vi "Accurate Measure_BU2.vi"(0 "DMM ref in":refnum<visa-resource-name>, 1 "channel_count":i32=11, 2 "P_current_count":i32, 3 "N_current_count":i32, 5 "DMM error in":errorcluster, 7 "Enable DMM-\nRelay":bool=TRUE, 9 "ESP32 ref in":refnum<visa-resource-name>, 11 "ESP32 error in":errorcluster, 12 "current_mode":u8[](array[numeric])=[0, 0, 0, 0, 0, 0, 0, 0, 0, 0, 0]) -> (4 "DMM ref out":refnum<visa-resource-name>, 6 "DMM error out":errorcluster, 8 "Accurate Data":dbl[](array[numeric]), 10 "ESP32 ref out":refnum<visa-resource-name>, 13 "time_out_count":i32, 14 "Standard Deviation of Data":dbl[](array[numeric]), 15 "ESP32 error out":errorcluster)   [LabVIEW 2023]
uses:
  <instrlib>/Agilent 3446X Series/Agilent 3446X Series.lvlib
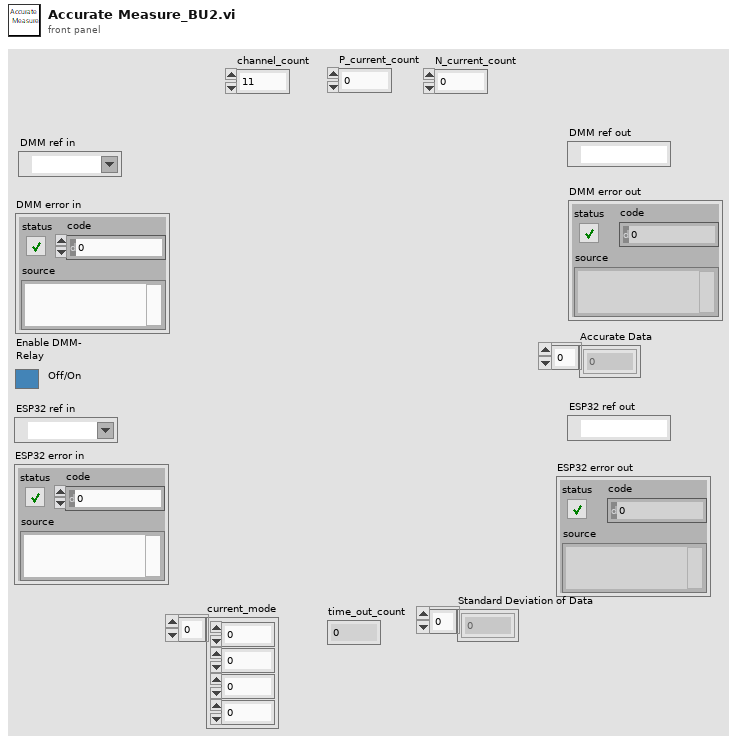
[diagram p1: front panel]
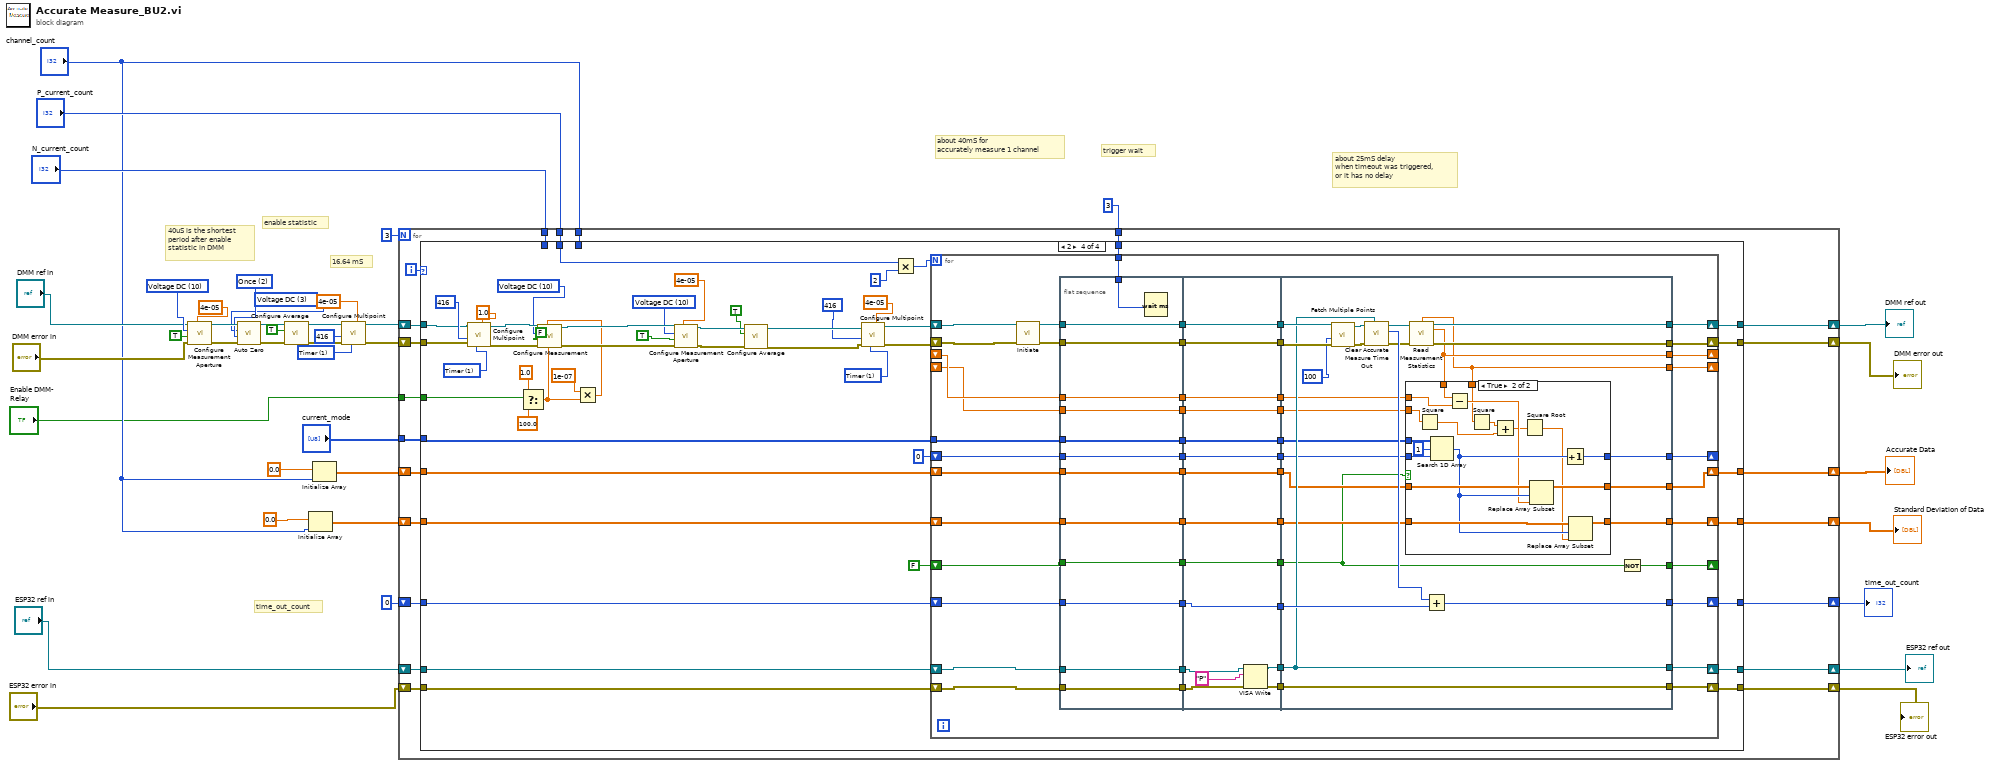
[diagram p0: block diagram]
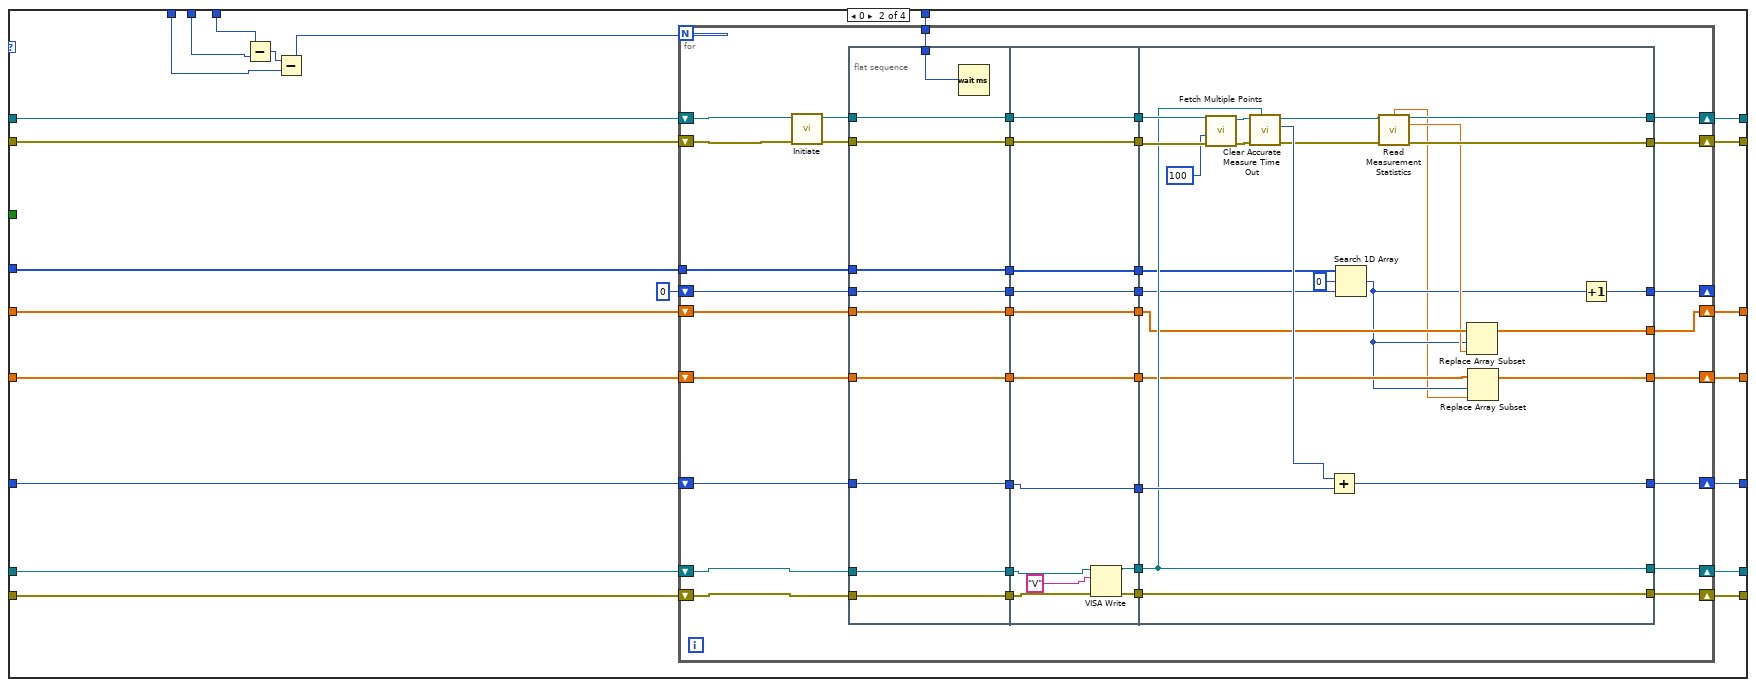
[diagram p3: hidden frame]
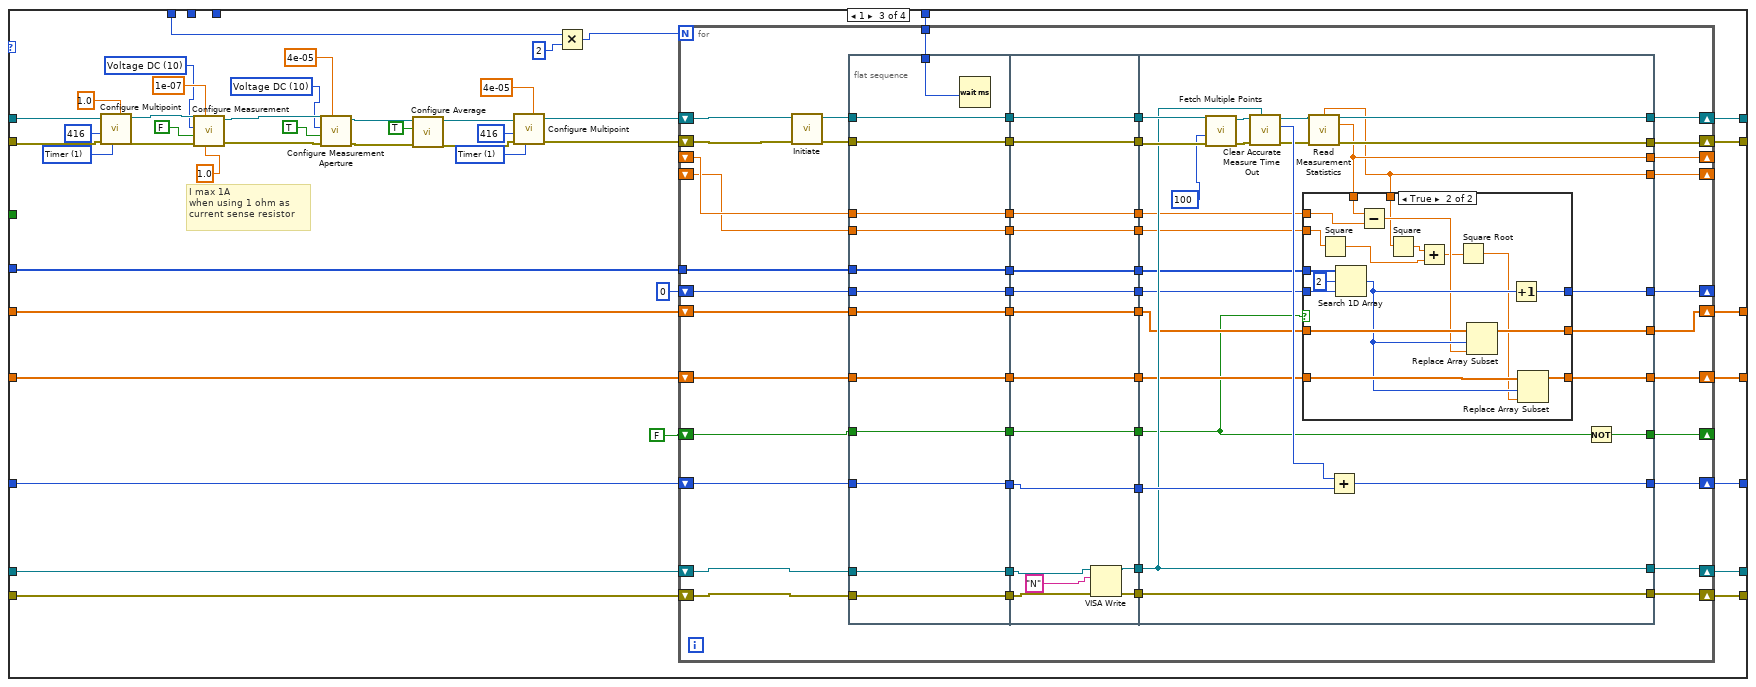
[diagram p4: hidden frame]
diagram:
  w27 = 1 items=["Immediate", "Timer"] ("Sample Source (0: Immediate)")
  w34 = 3 items=["Current DC", "Resistance", "Temperature", "Voltage DC"] ("Zero Type (0: Current DC)")
  w35 = 2 items=["Disable", "Enable", "Once"] ("Auto Zero (1: Enable)")
  w31 = 10 items=["Continuity", "Current AC", "Current DC", "Diode", "Frequency", "Resistance 4-wire", "Period", "Resistance 2-wire", "Temperature", "Voltage AC", "Voltage DC", "Voltage DC Ratio", "Capacitance"] ("Measurement Function (0: Continuity)")
  # "about 40mS for \naccurately measure 1 channel"
  # "about 25mS delay\nwhen timeout was triggered,\nor it has no delay"
  # "time_out_count"
  # "trigger wait"
  # "16.64 mS"
  # "enable statistic"
  # "40uS is the shortest\nperiod after enable \nstatistic in DMM"
  n1 = call <instrlib>:"Configure Measurement Aperture.vi"("Aperture Time (0.1s)"=4e-05, "error in (no error)"="DMM error in", "Enable Aperture (F: Disable)"=TRUE, "Measurement Function (0: Continuity)"=w31, "VISA resource name"="DMM ref in") -> ("error out"=w38:errorcluster, "VISA resource name out"=w37:refnum<visa-resource-name>)  [unwired: 5 in]
  n2 = call <instrlib>:"Auto Zero.vi"("error in (no error)"=w38, "Auto Zero (1: Enable)"=w35, "Zero Type (0: Current DC)"=w34, "VISA resource name"=w37) -> ("error out"=w40:errorcluster, "VISA resource name out"=w39:refnum<visa-resource-name>)  [unwired: 6 in]
  n3 = call <instrlib>:"Configure Average.vi"("error in (no error)"=w40, "Enable Statistics (F: Disable)"=TRUE, "VISA resource name"=w39) -> ("error out"=w29:errorcluster, "VISA resource name out"=w30:refnum<visa-resource-name>)  [unwired: 7 in]
  n4 = Initialize Array(0.0 ("Arithmetic Mean"), "channel_count") -> (w10:dbl[])
  n5 = Initialize Array(0.0 ("Arithmetic Mean"), "channel_count") -> (w13:dbl[])
  n6 = call <instrlib>:"Configure Multipoint.vi"("Sample Interval (1 Second)"=4e-05, "Sample Source (0: Immediate)"=w27, "error in (no error)"=w29, "Sample Count (1)"=416, "VISA resource name"=w30) -> ("error out"=w24:errorcluster, "VISA resource name out"=w25:refnum<visa-resource-name>)  [unwired: 2 in, 3 out]
  n7 = for {
    N: 3 -> [_]
    shift-right: [w59] -> w4
    shift-left: "ESP32 ref in" -> [w61]
    shift-right: [w58] -> w3
    shift-left: "ESP32 error in" -> [w60]
    shift-right: [w55] -> w6
    shift-left: w25 -> [w57]
    shift-right: [w54] -> w5
    shift-left: w24 -> [w56]
    tunnel: "channel_count" -> [w53]
    tunnel: "P_current_count" -> [w52]
    tunnel: "N_current_count" -> [w51]
    tunnel: u32 3 ("milliseconds to wait") -> [w50]
    shift-right: [w49] -> w15
    shift-left: 0 -> [w48]
    shift-right: [w42] -> w2
    shift-left: w13 -> [w47]
    tunnel: "current_mode" -> [w46]
    shift-right: [w43] -> w1
    shift-left: w10 -> [w44]
    tunnel: "Enable DMM-\nRelay" -> [w41]
    i -> [w45]
    n8 = case shown="2" w45 {
      tunnel: w61 -> [w66 w86 w220 w395]
      tunnel: w60 -> [w65 w85 w219 w394]
      tunnel: [w66 w82 w216 w391] -> w59
      tunnel: [w65 w81 w215 w390] -> w58
      tunnel: w57 -> [w68 w88 w182 w352]
      tunnel: w56 -> [w67 w87 w181 w351]
      tunnel: [w68 w84 w218 w393] -> w55
      tunnel: [w67 w83 w217 w392] -> w54
      tunnel: w53 -> [_ w80 _ _]
      tunnel: w52 -> [_ w79 _ w348]
      tunnel: w51 -> [_ w78 w177 _]
      tunnel: [w62 w76 w213 w388] -> w49
      tunnel: w50 -> [_ w77 w214 w389]
      tunnel: w48 -> [w62 w75 w212 w387]
      tunnel: w47 -> [w64 w73 w210 w385]
      tunnel: w46 -> [_ w74 w211 w386]
      tunnel: w44 -> [w63 w71 w208 w383]
      tunnel: [w63 w70 w207 w382] -> w43
      tunnel: [w64 w69 w206 w381] -> w42
      tunnel: w41 -> [_ _ _ w353]
      frame Default {
      }
      frame 0 {
        n9 = Subtract(x=w80, y=w79) -> (x-y=w90:i32)
        n10 = Subtract(x=w90, y=w78) -> (x-y=w89:i32)
        n11 = for {
          N: w89 -> [_]
          shift-right: [w124] -> w84
          shift-left: w88 -> [w128]
          shift-right: [w123] -> w83
          shift-left: w87 -> [w127]
          shift-right: [w122] -> w82
          shift-left: w86 -> [w126]
          shift-right: [w121] -> w81
          shift-left: w85 -> [w125]
          tunnel: w77 -> [w107]
          shift-right: [w106] -> w76
          shift-left: w75 -> [w120]
          tunnel: w74 -> [w104]
          shift-right: [w92] -> w69
          shift-left: w73 -> [w101]
          shift-right: [w96] -> _
          shift-left: 0 ("index of element") -> [w97]
          shift-right: [w91] -> w70
          shift-left: w71 -> [w94]
          n12 = call <instrlib>:"Initiate.vi"("error in (no error)"=w127, "VISA resource name"=w128) -> ("error out"=w108:errorcluster, "VISA resource name out"=w109:refnum<visa-resource-name>)  [unwired: 8 in]
          n13 = flat-sequence {
            tunnel: [w138] -> w119
            tunnel: w126 -> [w138]
            tunnel: [w137] -> w118
            tunnel: w125 -> [w137]
            tunnel: w109 -> [w136]
            tunnel: [w136] -> w117
            tunnel: [w135] -> w116
            tunnel: w108 -> [w135]
            tunnel: [w134] -> w115
            tunnel: w120 -> [w134]
            tunnel: w107 -> [w133]
            tunnel: [w132] -> w105
            tunnel: w104 -> [w132]
            tunnel: [w131] -> w102
            tunnel: w101 -> [w131]
            tunnel: w97 -> [w130]
            tunnel: [w130] -> w99
            tunnel: [w129] -> w95
            tunnel: w94 -> [w129]
            tunnel: w119 -> [w150]
            tunnel: w118 -> [w149]
            tunnel: w117 -> [w148]
            tunnel: [w148] -> w111
            tunnel: w116 -> [w147]
            tunnel: [w147] -> w112
            tunnel: [w146] -> w113
            tunnel: [w145] -> w114
            tunnel: w115 -> [w143]
            tunnel: [w143] -> w110
            tunnel: w105 -> [w142]
            tunnel: [w142] -> w103
            tunnel: w102 -> [w141]
            tunnel: [w141] -> w100
            tunnel: w99 -> [w140]
            tunnel: [w140] -> w98
            tunnel: w95 -> [w139]
            tunnel: [w139] -> w93
            tunnel: [w175] -> w121
            tunnel: [w163] -> w122
            tunnel: [w167] -> w123
            tunnel: [w168] -> w124
            tunnel: w114 -> [w175]
            tunnel: w113 -> [w163]
            tunnel: w112 -> [w174]
            tunnel: w111 -> [w173]
            tunnel: [w169] -> w106
            tunnel: w110 -> [w164]
            tunnel: w103 -> [w162]
            tunnel: w100 -> [w158]
            tunnel: w98 -> [w160]
            tunnel: [w159] -> w96
            tunnel: w93 -> [w156]
            tunnel: [w153] -> w92
            tunnel: [w152] -> w91
            frame #0 {
              n14 = Wait (ms)(milliseconds to wait=w133) -> ()  [unwired: 1 out]
            }
            frame #1 {
              n15 = VISA Write(VISA resource name=w150, write buffer="V" ("data in"), error in (no error)=w149) -> (VISA resource name out=w146:refnum<visa-resource-name>, error out=w145:errorcluster)  [unwired: 1 out]
            }
            frame #2 {
              n16 = call <instrlib>:"Fetch Multiple Points.vi"("error in (no error)"=w174, "Timeout (10000 ms)"=100, "VISA resource name"=w173) -> ("error out"=w171:errorcluster, "VISA resource name out"=w172:refnum<visa-resource-name>)  [unwired: 1 in, 6 out]
              n17 = call "Clear Accurate Measure Time Out.vi"("ESP32 ref"=w163, "error in (no error)"=w171, "DMM ref"=w172) -> ("error out"=w165:errorcluster, "Time out count"=w170:i32, "VISA Refnum out"=w166:refnum<visa-resource-name>)  [unwired: 5 in, 1 out]
              n18 = Add(x=w170, y=w164) -> (x+y=w169:i32)
              n19 = Search 1D Array(1D array=w162, element=u8 0, start index (0)=w160) -> (index of element=w155:i32)
              n20 = call <instrlib>:"Read Measurement Statistics.vi"("VISA resource name"=w166, "error in (no error)"=w165) -> ("Standard Deviation"=w154:dbl, "VISA resource name out"=w168:refnum<visa-resource-name>, "Arithmetic Mean"=w157:dbl, "error out"=w167:errorcluster)  [unwired: 6 in, 4 out]
              n21 = Replace Array Subset(array=w158, new element=w157, index=w155) -> (w153:dbl[])
              n22 = Replace Array Subset(array=w156, new element=w154, index=w155) -> (w152:dbl[])
              n23 = Increment(x=w155) -> (x+1=w159:i32)
            }
          }
        }
      }
      frame 1 {
        w195 = 1 items=["Immediate", "Timer"] ("Sample Source (0: Immediate)")
        w191 = 10 items=["Continuity", "Current AC", "Current DC", "Diode", "Frequency", "Resistance 4-wire", "Period", "Resistance 2-wire", "Temperature", "Voltage AC", "Voltage DC", "Voltage DC Ratio", "Capacitance"] ("Measurement Function (0: Continuity)")
        w188 = 1 items=["Immediate", "Timer"] ("Sample Source (0: Immediate)")
        w183 = 10 items=["Continuity", "Current AC", "Current DC", "Diode", "Frequency", "Resistance 4-wire", "Period", "Resistance 2-wire", "Temperature", "Voltage AC", "Voltage DC", "Voltage DC Ratio", "Capacitance"] ("Measurement Function (10: Voltage DC)")
        # "I max 1A\nwhen using 1 ohm as \ncurrent sense resistor"
        n24 = call <instrlib>:"Configure Multipoint.vi"("Sample Interval (1 Second)"=1.0, "Sample Source (0: Immediate)"=w188, "error in (no error)"=w181, "Sample Count (1)"=416, "VISA resource name"=w182) -> ("error out"=w202:errorcluster, "VISA resource name out"=w201:refnum<visa-resource-name>)  [unwired: 2 in, 3 out]
        n25 = call <instrlib>:"Configure Measurement.vi"("Manual Range (1)"=1.0, "Absolute Resolution (1E-6)"=1e-07, "error in (no error)"=w202, "Auto Range (T: Enable)"=FALSE, "Measurement Function (10: Voltage DC)"=w183, "VISA resource name"=w201) -> ("error out"=w199:errorcluster, "VISA resource name out"=w200:refnum<visa-resource-name>)  [unwired: 4 out]
        n26 = call <instrlib>:"Configure Measurement Aperture.vi"("Aperture Time (0.1s)"=4e-05, "error in (no error)"=w199, "Enable Aperture (F: Disable)"=TRUE, "Measurement Function (0: Continuity)"=w191, "VISA resource name"=w200) -> ("error out"=w204:errorcluster, "VISA resource name out"=w205:refnum<visa-resource-name>)  [unwired: 5 in]
        n27 = call <instrlib>:"Configure Average.vi"("error in (no error)"=w204, "Enable Statistics (F: Disable)"=TRUE, "VISA resource name"=w205) -> ("error out"=w203:errorcluster, "VISA resource name out"=w198:refnum<visa-resource-name>)  [unwired: 7 in]
        n28 = call <instrlib>:"Configure Multipoint.vi"("Sample Interval (1 Second)"=4e-05, "Sample Source (0: Immediate)"=w195, "error in (no error)"=w203, "Sample Count (1)"=416, "VISA resource name"=w198) -> ("error out"=w179:errorcluster, "VISA resource name out"=w180:refnum<visa-resource-name>)  [unwired: 2 in, 3 out]
        n29 = Multiply(x=w177, y=2) -> (x*y=w178:i32)
        n30 = for {
          N: w178 -> [_]
          shift-right: [w266] -> w218
          shift-left: w180 -> [w270]
          shift-right: [w265] -> w217
          shift-left: w179 -> [w269]
          shift-right: [w264] -> w216
          shift-left: w220 -> [w268]
          shift-right: [w263] -> w215
          shift-left: w219 -> [w267]
          tunnel: w214 -> [w249]
          shift-right: [w248] -> w213
          shift-left: w212 -> [w262]
          tunnel: w211 -> [w246]
          shift-right: [w234] -> w206
          shift-left: w210 -> [w243]
          shift-right: [w238] -> _
          shift-left: 0 ("index of element") -> [w239]
          shift-right: [w233] -> w207
          shift-left: w208 -> [w236]
          shift-right: [w229] -> _
          shift-left: FALSE ("Enable Statistics (F: Disable)") -> [w230]
          shift-right: [w228] -> _
          shift-left: _ -> [w226]
          shift-right: [w227] -> _
          shift-left: _ -> [w223]
          n31 = call <instrlib>:"Initiate.vi"("error in (no error)"=w269, "VISA resource name"=w270) -> ("error out"=w250:errorcluster, "VISA resource name out"=w251:refnum<visa-resource-name>)  [unwired: 8 in]
          n32 = flat-sequence {
            tunnel: [w283] -> w261
            tunnel: w268 -> [w283]
            tunnel: [w282] -> w260
            tunnel: w267 -> [w282]
            tunnel: w251 -> [w281]
            tunnel: [w281] -> w259
            tunnel: [w280] -> w258
            tunnel: w250 -> [w280]
            tunnel: [w279] -> w257
            tunnel: w262 -> [w279]
            tunnel: w249 -> [w278]
            tunnel: [w277] -> w247
            tunnel: w246 -> [w277]
            tunnel: [w276] -> w244
            tunnel: w243 -> [w276]
            tunnel: w239 -> [w275]
            tunnel: [w275] -> w241
            tunnel: [w274] -> w237
            tunnel: w236 -> [w274]
            tunnel: w230 -> [w273]
            tunnel: [w273] -> w232
            tunnel: w226 -> [w272]
            tunnel: [w272] -> w224
            tunnel: w223 -> [w271]
            tunnel: [w271] -> w222
            tunnel: w261 -> [w298]
            tunnel: w260 -> [w297]
            tunnel: w259 -> [w296]
            tunnel: [w296] -> w253
            tunnel: w258 -> [w295]
            tunnel: [w295] -> w254
            tunnel: [w294] -> w255
            tunnel: [w293] -> w256
            tunnel: w257 -> [w291]
            tunnel: [w291] -> w252
            tunnel: w247 -> [w290]
            tunnel: [w290] -> w245
            tunnel: w244 -> [w289]
            tunnel: [w289] -> w242
            tunnel: w241 -> [w288]
            tunnel: [w288] -> w240
            tunnel: w237 -> [w287]
            tunnel: [w287] -> w235
            tunnel: w232 -> [w286]
            tunnel: [w286] -> w231
            tunnel: [w285] -> w225
            tunnel: w224 -> [w285]
            tunnel: w222 -> [w284]
            tunnel: [w284] -> w221
            tunnel: [w325] -> w263
            tunnel: [w313] -> w264
            tunnel: [w317] -> w265
            tunnel: [w318] -> w266
            tunnel: w256 -> [w325]
            tunnel: w255 -> [w313]
            tunnel: w254 -> [w324]
            tunnel: w253 -> [w323]
            tunnel: [w319] -> w248
            tunnel: w252 -> [w314]
            tunnel: w245 -> [w312]
            tunnel: w242 -> [w309]
            tunnel: w240 -> [w311]
            tunnel: [w310] -> w238
            tunnel: w235 -> [w308]
            tunnel: [w307] -> w234
            tunnel: [w306] -> w233
            tunnel: w231 -> [w305]
            tunnel: [w304] -> w229
            tunnel: [w301] -> w228
            tunnel: [w300] -> w227
            tunnel: w225 -> [w303]
            tunnel: w221 -> [w302]
            frame #0 {
              n33 = Wait (ms)(milliseconds to wait=w278) -> ()  [unwired: 1 out]
            }
            frame #1 {
              n34 = VISA Write(VISA resource name=w298, write buffer="N" ("data in"), error in (no error)=w297) -> (VISA resource name out=w294:refnum<visa-resource-name>, error out=w293:errorcluster)  [unwired: 1 out]
            }
            frame #2 {
              n35 = call <instrlib>:"Fetch Multiple Points.vi"("error in (no error)"=w324, "Timeout (10000 ms)"=100, "VISA resource name"=w323) -> ("error out"=w321:errorcluster, "VISA resource name out"=w322:refnum<visa-resource-name>)  [unwired: 1 in, 6 out]
              n36 = call "Clear Accurate Measure Time Out.vi"("ESP32 ref"=w313, "error in (no error)"=w321, "DMM ref"=w322) -> ("error out"=w315:errorcluster, "Time out count"=w320:i32, "VISA Refnum out"=w316:refnum<visa-resource-name>)  [unwired: 5 in, 1 out]
              n37 = call <instrlib>:"Read Measurement Statistics.vi"("VISA resource name"=w316, "error in (no error)"=w315) -> ("Standard Deviation"=w300:dbl, "VISA resource name out"=w318:refnum<visa-resource-name>, "Arithmetic Mean"=w301:dbl, "error out"=w317:errorcluster)  [unwired: 6 in, 4 out]
              n38 = case shown="True" w305 {
                tunnel: w312 -> [_ w346]
                tunnel: w311 -> [w328 w344]
                tunnel: [w328 w343] -> w310
                tunnel: w309 -> [w327 w342]
                tunnel: w308 -> [w326 w341]
                tunnel: [w327 w339] -> w307
                tunnel: [w326 w338] -> w306
                tunnel: w303 -> [_ w329]
                tunnel: w302 -> [_ w336]
                tunnel: w301 -> [_ w330]
                tunnel: w300 -> [_ w335]
                frame False {
                }
                frame True {
                  n39 = Square(x=w336) -> (x^2=w333:dbl)
                  n40 = Search 1D Array(1D array=w346, element=u8 2, start index (0)=w344) -> (index of element=w340:i32)
                  n41 = Subtract(x=w330, y=w329) -> (x-y=w337:dbl)
                  n42 = Square(x=w335) -> (x^2=w334:dbl)
                  n43 = Add(x=w334, y=w333) -> (x+y=w332:dbl)
                  n44 = Square Root(x=w332) -> (sqrt(x)=w331:dbl)
                  n45 = Replace Array Subset(array=w342, new element=w337, index=w340) -> (w339:dbl[])
                  n46 = Increment(x=w340) -> (x+1=w343:i32)
                  n47 = Replace Array Subset(array=w341, new element=w331, index=w340) -> (w338:dbl[])
                }
              }
              n48 = Add(x=w320, y=w314) -> (x+y=w319:i32)
              n49 = Not(x=w305) -> (.not. x?=w304:bool)
            }
          }
        }
      }
      frame 2 {
        w367 = 1 items=["Immediate", "Timer"] ("Sample Source (0: Immediate)")
        w363 = 10 items=["Continuity", "Current AC", "Current DC", "Diode", "Frequency", "Resistance 4-wire", "Period", "Resistance 2-wire", "Temperature", "Voltage AC", "Voltage DC", "Voltage DC Ratio", "Capacitance"] ("Measurement Function (0: Continuity)")
        w360 = 1 items=["Immediate", "Timer"] ("Sample Source (0: Immediate)")
        w357 = 10 items=["Continuity", "Current AC", "Current DC", "Diode", "Frequency", "Resistance 4-wire", "Period", "Resistance 2-wire", "Temperature", "Voltage AC", "Voltage DC", "Voltage DC Ratio", "Capacitance"] ("Measurement Function (10: Voltage DC)")
        n50 = call <instrlib>:"Configure Multipoint.vi"("Sample Interval (1 Second)"=1.0, "Sample Source (0: Immediate)"=w360, "error in (no error)"=w351, "Sample Count (1)"=416, "VISA resource name"=w352) -> ("error out"=w376:errorcluster, "VISA resource name out"=w375:refnum<visa-resource-name>)  [unwired: 2 in, 3 out]
        n51 = Select(t=1.0 ("Manual Range (1)"), s=w353, f=100.0 ("Manual Range (1)")) -> (s? t:f=w356:dbl)
        n52 = Multiply(x=1e-07, y=w356) -> (x*y=w355:dbl)
        n53 = call <instrlib>:"Configure Measurement.vi"("Manual Range (1)"=w356, "Absolute Resolution (1E-6)"=w355, "error in (no error)"=w376, "Auto Range (T: Enable)"=FALSE, "Measurement Function (10: Voltage DC)"=w357, "VISA resource name"=w375) -> ("error out"=w373:errorcluster, "VISA resource name out"=w374:refnum<visa-resource-name>)  [unwired: 4 out]
        n54 = call <instrlib>:"Configure Measurement Aperture.vi"("Aperture Time (0.1s)"=4e-05, "error in (no error)"=w373, "Enable Aperture (F: Disable)"=TRUE, "Measurement Function (0: Continuity)"=w363, "VISA resource name"=w374) -> ("error out"=w378:errorcluster, "VISA resource name out"=w379:refnum<visa-resource-name>)  [unwired: 5 in]
        n55 = call <instrlib>:"Configure Average.vi"("error in (no error)"=w378, "Enable Statistics (F: Disable)"=TRUE, "VISA resource name"=w379) -> ("error out"=w377:errorcluster, "VISA resource name out"=w372:refnum<visa-resource-name>)  [unwired: 7 in]
        n56 = call <instrlib>:"Configure Multipoint.vi"("Sample Interval (1 Second)"=4e-05, "Sample Source (0: Immediate)"=w367, "error in (no error)"=w377, "Sample Count (1)"=416, "VISA resource name"=w372) -> ("error out"=w349:errorcluster, "VISA resource name out"=w350:refnum<visa-resource-name>)  [unwired: 2 in, 3 out]
        n57 = Multiply(x=w348, y=2) -> (x*y=w347:i32)
        n58 = for {
          N: w347 -> [_]
          shift-right: [w441] -> w393
          shift-left: w350 -> [w445]
          shift-right: [w440] -> w392
          shift-left: w349 -> [w444]
          shift-right: [w439] -> w391
          shift-left: w395 -> [w443]
          shift-right: [w438] -> w390
          shift-left: w394 -> [w442]
          tunnel: w389 -> [w424]
          shift-right: [w423] -> w388
          shift-left: w387 -> [w437]
          tunnel: w386 -> [w421]
          shift-right: [w409] -> w381
          shift-left: w385 -> [w418]
          shift-right: [w413] -> _
          shift-left: 0 ("index of element") -> [w414]
          shift-right: [w408] -> w382
          shift-left: w383 -> [w411]
          shift-right: [w404] -> _
          shift-left: FALSE ("Enable Statistics (F: Disable)") -> [w405]
          shift-right: [w403] -> _
          shift-left: _ -> [w401]
          shift-right: [w402] -> _
          shift-left: _ -> [w398]
          n59 = call <instrlib>:"Initiate.vi"("error in (no error)"=w444, "VISA resource name"=w445) -> ("error out"=w425:errorcluster, "VISA resource name out"=w426:refnum<visa-resource-name>)  [unwired: 8 in]
          n60 = flat-sequence {
            tunnel: [w458] -> w436
            tunnel: w443 -> [w458]
            tunnel: [w457] -> w435
            tunnel: w442 -> [w457]
            tunnel: w426 -> [w456]
            tunnel: [w456] -> w434
            tunnel: [w455] -> w433
            tunnel: w425 -> [w455]
            tunnel: [w454] -> w432
            tunnel: w437 -> [w454]
            tunnel: w424 -> [w453]
            tunnel: [w452] -> w422
            tunnel: w421 -> [w452]
            tunnel: [w451] -> w419
            tunnel: w418 -> [w451]
            tunnel: w414 -> [w450]
            tunnel: [w450] -> w416
            tunnel: [w449] -> w412
            tunnel: w411 -> [w449]
            tunnel: w405 -> [w448]
            tunnel: [w448] -> w407
            tunnel: w401 -> [w447]
            tunnel: [w447] -> w399
            tunnel: w398 -> [w446]
            tunnel: [w446] -> w397
            tunnel: w436 -> [w473]
            tunnel: w435 -> [w472]
            tunnel: w434 -> [w471]
            tunnel: [w471] -> w428
            tunnel: w433 -> [w470]
            tunnel: [w470] -> w429
            tunnel: [w469] -> w430
            tunnel: [w468] -> w431
            tunnel: w432 -> [w466]
            tunnel: [w466] -> w427
            tunnel: w422 -> [w465]
            tunnel: [w465] -> w420
            tunnel: w419 -> [w464]
            tunnel: [w464] -> w417
            tunnel: w416 -> [w463]
            tunnel: [w463] -> w415
            tunnel: w412 -> [w462]
            tunnel: [w462] -> w410
            tunnel: w407 -> [w461]
            tunnel: [w461] -> w406
            tunnel: [w460] -> w400
            tunnel: w399 -> [w460]
            tunnel: w397 -> [w459]
            tunnel: [w459] -> w396
            tunnel: [w500] -> w438
            tunnel: [w488] -> w439
            tunnel: [w492] -> w440
            tunnel: [w493] -> w441
            tunnel: w431 -> [w500]
            tunnel: w430 -> [w488]
            tunnel: w429 -> [w499]
            tunnel: w428 -> [w498]
            tunnel: [w494] -> w423
            tunnel: w427 -> [w489]
            tunnel: w420 -> [w487]
            tunnel: w417 -> [w484]
            tunnel: w415 -> [w486]
            tunnel: [w485] -> w413
            tunnel: w410 -> [w483]
            tunnel: [w482] -> w409
            tunnel: [w481] -> w408
            tunnel: w406 -> [w480]
            tunnel: [w479] -> w404
            tunnel: [w476] -> w403
            tunnel: [w475] -> w402
            tunnel: w400 -> [w478]
            tunnel: w396 -> [w477]
            frame #0 {
              n61 = Wait (ms)(milliseconds to wait=w453) -> ()  [unwired: 1 out]
            }
            frame #1 {
              n62 = VISA Write(VISA resource name=w473, write buffer="P" ("data in"), error in (no error)=w472) -> (VISA resource name out=w469:refnum<visa-resource-name>, error out=w468:errorcluster)  [unwired: 1 out]
            }
            frame #2 {
              n63 = call <instrlib>:"Fetch Multiple Points.vi"("error in (no error)"=w499, "Timeout (10000 ms)"=100, "VISA resource name"=w498) -> ("error out"=w496:errorcluster, "VISA resource name out"=w497:refnum<visa-resource-name>)  [unwired: 1 in, 6 out]
              n64 = call "Clear Accurate Measure Time Out.vi"("ESP32 ref"=w488, "error in (no error)"=w496, "DMM ref"=w497) -> ("error out"=w490:errorcluster, "Time out count"=w495:i32, "VISA Refnum out"=w491:refnum<visa-resource-name>)  [unwired: 5 in, 1 out]
              n65 = call <instrlib>:"Read Measurement Statistics.vi"("VISA resource name"=w491, "error in (no error)"=w490) -> ("Standard Deviation"=w475:dbl, "VISA resource name out"=w493:refnum<visa-resource-name>, "Arithmetic Mean"=w476:dbl, "error out"=w492:errorcluster)  [unwired: 6 in, 4 out]
              n66 = case shown="True" w480 {
                tunnel: w487 -> [_ w521]
                tunnel: w486 -> [w503 w519]
                tunnel: [w503 w518] -> w485
                tunnel: w484 -> [w502 w517]
                tunnel: w483 -> [w501 w516]
                tunnel: [w502 w514] -> w482
                tunnel: [w501 w513] -> w481
                tunnel: w478 -> [_ w504]
                tunnel: w477 -> [_ w511]
                tunnel: w476 -> [_ w505]
                tunnel: w475 -> [_ w510]
                frame False {
                }
                frame True {
                  n67 = Square(x=w511) -> (x^2=w508:dbl)
                  n68 = Search 1D Array(1D array=w521, element=u8 1, start index (0)=w519) -> (index of element=w515:i32)
                  n69 = Subtract(x=w505, y=w504) -> (x-y=w512:dbl)
                  n70 = Square(x=w510) -> (x^2=w509:dbl)
                  n71 = Add(x=w509, y=w508) -> (x+y=w507:dbl)
                  n72 = Square Root(x=w507) -> (sqrt(x)=w506:dbl)
                  n73 = Replace Array Subset(array=w517, new element=w512, index=w515) -> (w514:dbl[])
                  n74 = Increment(x=w515) -> (x+1=w518:i32)
                  n75 = Replace Array Subset(array=w516, new element=w506, index=w515) -> (w513:dbl[])
                }
              }
              n76 = Add(x=w495, y=w489) -> (x+y=w494:i32)
              n77 = Not(x=w480) -> (.not. x?=w479:bool)
            }
          }
        }
      }
    }
  }
  "time_out_count" <- w15
  "DMM ref out" <- w6
  "DMM error out" <- w5
  "ESP32 ref out" <- w4
  "ESP32 error out" <- w3
  "Accurate Data" <- w2
  "Standard Deviation of Data" <- w1
